vi "frame-capture.vi"() -> ()   [LabVIEW 2012]
uses:
  <vilib>/DAQmx/create/channels.llb/DAQmx Create Channel (AI-Voltage-Basic).vi
  <vilib>/DAQmx/create/channels.llb/DAQmx Create Channel (DO-Digital Output).vi
  <vilib>/DAQmx/create/channels.llb/DAQmx Create Channel (AO-Voltage-Basic).vi
  <vilib>/DAQmx/write.llb/DAQmx Write (Digital Bool 1Line 1Point).vi
  <vilib>/DAQmx/configure/timing.llb/DAQmx Timing (Sample Clock).vi
  <vilib>/DAQmx/configure/trigger.llb/DAQmx Start Trigger (Digital Edge).vi
  <vilib>/DAQmx/write.llb/DAQmx Write (Analog 1D Wfm NChan NSamp).vi
panel:
  in  "Position Pin":tag="Dev1/ao0:1"
  in  "Read Pin":tag="Dev1/ai0"
  in  "Enable Pin":tag="Dev1/port0/line0"
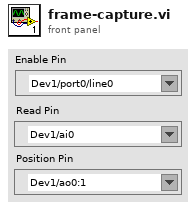
[diagram p1: front panel]
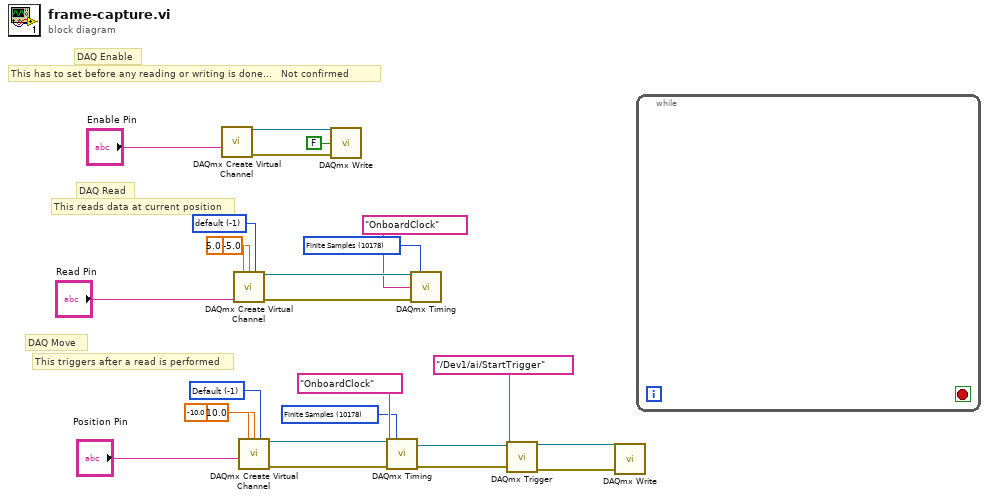
[diagram p0: block diagram]
diagram:
  w1 = 10178 items=["Finite Samples"=10178, "Continuous Samples"=10123, "Hardware Timed Single Point"=12522] ("sample mode")
  w2 = 10178 items=["Finite Samples"=10178, "Continuous Samples"=10123, "Hardware Timed Single Point"=12522] ("sample mode")
  w14 = -1 items=["Default"=-1, "RSE"=10083, "Differential"=10106, "Pseudodifferential"=12529] ("output terminal configuration")
  w18 = -1 items=["default"=-1, "RSE"=10083, "NRSE"=10078, "Differential"=10106, "Pseudodifferential"=12529] ("input terminal configuration")
  # "This has to set before any reading or writing is done...   Not confirmed"
  # "This triggers after a read is performed"
  # "This reads data at current position"
  # "DAQ Enable"
  # "DAQ Move"
  # "DAQ Read"
  n1 = call-poly <vilib>:"DAQmx Create Virtual Channel.vi"("lines"="Enable Pin") -> ("task out"=w21:refnum<k21>, "error out"=w22:errorcluster)  [unwired: 13 in]
  n2 = call-poly <vilib>:"DAQmx Create Virtual Channel.vi"("maximum value"=5.0, "minimum value"=-5.0, "input terminal configuration"=w18, "physical channels"="Read Pin") -> ("task out"=w10:refnum<k21>, "error out"=w11:errorcluster)  [unwired: 10 in]
  n3 = call-poly <vilib>:"DAQmx Create Virtual Channel.vi"("maximum value"=10.0, "minimum value"=-10.0, "output terminal configuration"=w14, "physical channels"="Position Pin") -> ("task out"=w12:refnum<k21>, "error out"=w13:errorcluster)  [unwired: 10 in]
  n4 = call-poly <vilib>:"DAQmx Write.vi"("task/channels in"=w21, "data"=FALSE, "error in"=w22) -> ()  [unwired: 10 in, 3 out]
  n5 = call-poly <vilib>:"DAQmx Timing.vi"("task/channels in"=w12, "sample mode"=w2, "source"=tag "OnboardClock", "error in"=w13) -> ("task out"=w8:refnum<k21>, "error out"=w9:errorcluster)  [unwired: 10 in]
  n6 = call-poly <vilib>:"DAQmx Timing.vi"("task/channels in"=w10, "sample mode"=w1, "source"=tag "OnboardClock", "error in"=w11) -> ()  [unwired: 10 in, 2 out]
  n7 = call-poly <vilib>:"DAQmx Trigger.vi"("task/channels in"=w8, "source"=tag "/Dev1/ai/StartTrigger", "error in"=w9) -> ("task out"=w6:refnum<k21>, "error out"=w7:errorcluster)  [unwired: 11 in]
  n8 = call-poly <vilib>:"DAQmx Write.vi"("task/channels in"=w6, "error in"=w7) -> ()  [unwired: 11 in, 3 out]
  n9 = while {
    stop <- _ stop-if-true
  }
